vi "Read By Message (Resp-StrArray).vi"(7 "Current Module (\"\" to Generate an ID)":string, 8 "error in (no error)":errorcluster, 9 "CSM Name":string, 10 "Arguments (\"\")":string, 11 "State":string="Python: List API") -> (0 "error out":errorcluster, 2 "Value":string[](array[string]))   [LabVIEW 2017, in "CSM-Helper.lvclass"]
doc: "### Read States.vi\n\n-- <b>Controls</b> --\n- <b>CSM-Helper in</b>: CSMHelper input\n\n-- <b>Indicators</b> --\n- <b>Value</b>:\n- <b>CSM-Helper out</b>: CSMHelper output"
uses:
  CSM-Helper.lvclass
  Communicable State Machine.lvlib
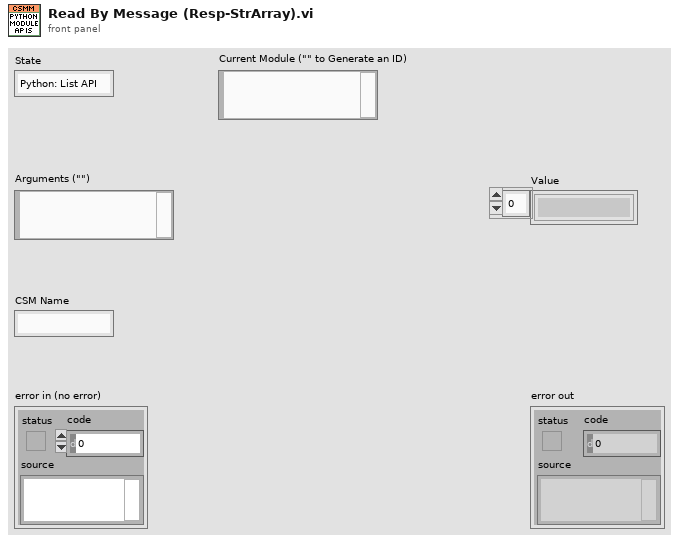
[diagram p1: front panel]
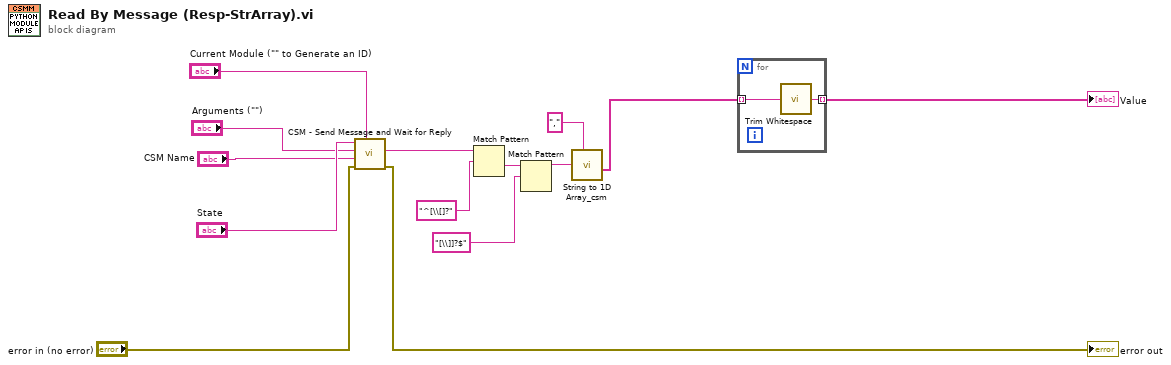
[diagram p0: block diagram]
diagram:
  n1 = call "CSM - Send Message and Wait for Reply.vi"("Current Module (\"\" to Generate an ID)"="Current Module (\"\" to Generate an ID)", "Error In (No Error)"="error in (no error)", "Target Module"="CSM Name", "Arguments (\"\")"="Arguments (\"\")", "State"="State") -> ("error out"=→"error out":errorcluster, "Response"=w13:string)  [unwired: 4 in, 1 out]
  n2 = Match Pattern(string=w13, regular expression="^[\\[]?" ("State")) -> (after substring=w12:string)  [unwired: 1 in, 3 out]
  n3 = Match Pattern(string=w12, regular expression="[\\]]?$" ("State")) -> (before substring=w11:string)  [unwired: 1 in, 3 out]
  n4 = call "String to 1D Array_csm.vi"("delimiter (Tab)"=",", "string"=w11) -> ("Array of Strings"=w7:string[])  [unwired: 9 in]
  n5 = for {
    tunnel: w7 -> [w16] mode=indexing
    tunnel: [w15] -> w6 mode=indexing
    n6 = call <vilib>:"Trim Whitespace.vi"("string"=w16) -> ("trimmed string"=w15:string)  [unwired: 1 in]
  }
  "Value" <- w6
